vi "GetParam.vi"(8 "error in (no error)":errorcluster caption="entrée d'erreur (pas d'erreur)", 11 "Linear_kernel.lvclass":refnum<class "Linear_kernel.lvclass">) -> (0 "error out":errorcluster caption="sortie d'erreur", 2 "linear_kernel":cluster{"dense_output":bool}={"dense_output"=TRUE}, 3 "Linear_kernel.lvclass":refnum<class "Linear_kernel.lvclass">)   [LabVIEW 2020, in "Linear_kernel.lvclass"]
doc: "Get Parameters"
uses:
  Linear_kernel.lvclass
  Linear_kernel.lvclass/Linear_kernel.ctl
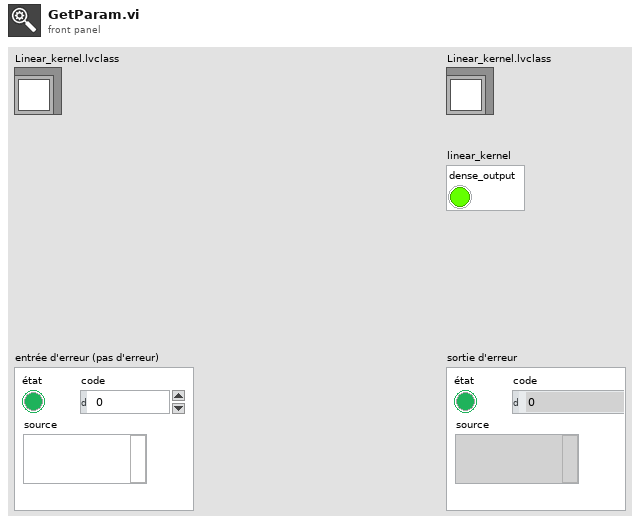
[diagram p1: front panel]
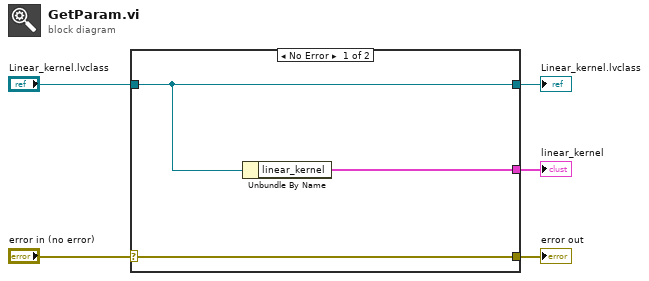
[diagram p0: block diagram]
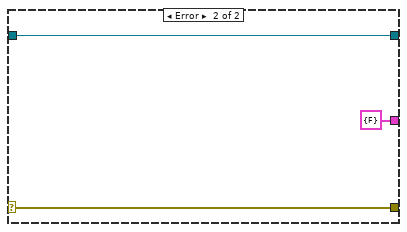
[diagram p2: hidden frame]
diagram:
  n1 = case shown="No Error" "error in (no error)" {
    selector: "error in (no error)" -> [w8 w10]
    tunnel: [w8 w10] -> w4
    tunnel: [w7 w11] -> w2
    tunnel: "Linear_kernel.lvclass" -> [w7 w11]
    tunnel: [w6 cluster{"dense_output":bool} {"dense_output"=FALSE} ("linear_kernel")] -> w1
    frame No Error {
      n2 = Unbundle By Name(w7) -> ("linear_kernel"=w6:cluster{"dense_output":bool})
    }
    frame Error {
    }
  }
  "error out" <- w4
  "Linear_kernel.lvclass" <- w2
  "linear_kernel" <- w1
